vi "Write Instrument ID.vi"(8 "error in (no error)":errorcluster, 10 "Instrument ID":u32, 11 "Instrument Data in":refnum<class "Instrument Data.lvclass">) -> (0 "error out":errorcluster, 3 "Instrument Data out":refnum<class "Instrument Data.lvclass">)   [LabVIEW 2020, in "Instrument Handler.lvlib" / "Instrument Data.lvclass"]
doc: "Write the 'Instrument ID' to the class private data."
uses:
  Instrument Data.lvclass
  Instrument Data.lvclass/Instrument Data.ctl
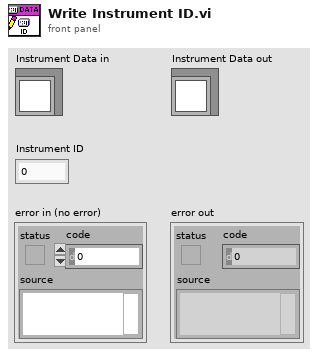
[diagram p1: front panel]
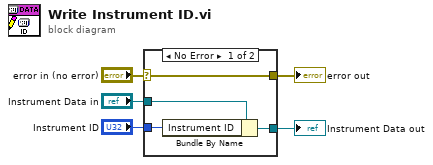
[diagram p0: block diagram]
diagram:
  n1 = case shown="No Error" "error in (no error)" {
    selector: "error in (no error)" -> [w9 w10]
    tunnel: [w9 w10] -> w4
    tunnel: [w7 w11] -> w2
    tunnel: "Instrument Data in" -> [w8 w11]
    tunnel: "Instrument ID" -> [w6 _]
    frame No Error {
      n2 = Bundle By Name(cluster=w8, "Instrument ID"=w6) -> (w7:refnum<class "Instrument Data.lvclass">)
    }
    frame Error {
    }
  }
  "error out" <- w4
  "Instrument Data out" <- w2
